vi "VFH-comp-libreVNAR140.vi"() -> ()   [LabVIEW 2020, in "VFH-VNA_File_Handler.lvlib"]
uses:
  VFH-VNA_File_Handler.lvlib
panel:
  out "Waveform Graph":dbl[][](graph)
  out "Raw 2":T1(graph)
  in  "r140":path=path "C:/projects/UNI/VNA/MiniVNA/20240625-162312-Vann/Vann.txt"
  out "Raw":T1(graph)
  in  "Libre":path=path "C:/projects/UNI/VNA/MiniVNA/20240625-162312-Vann/Vann.txt"
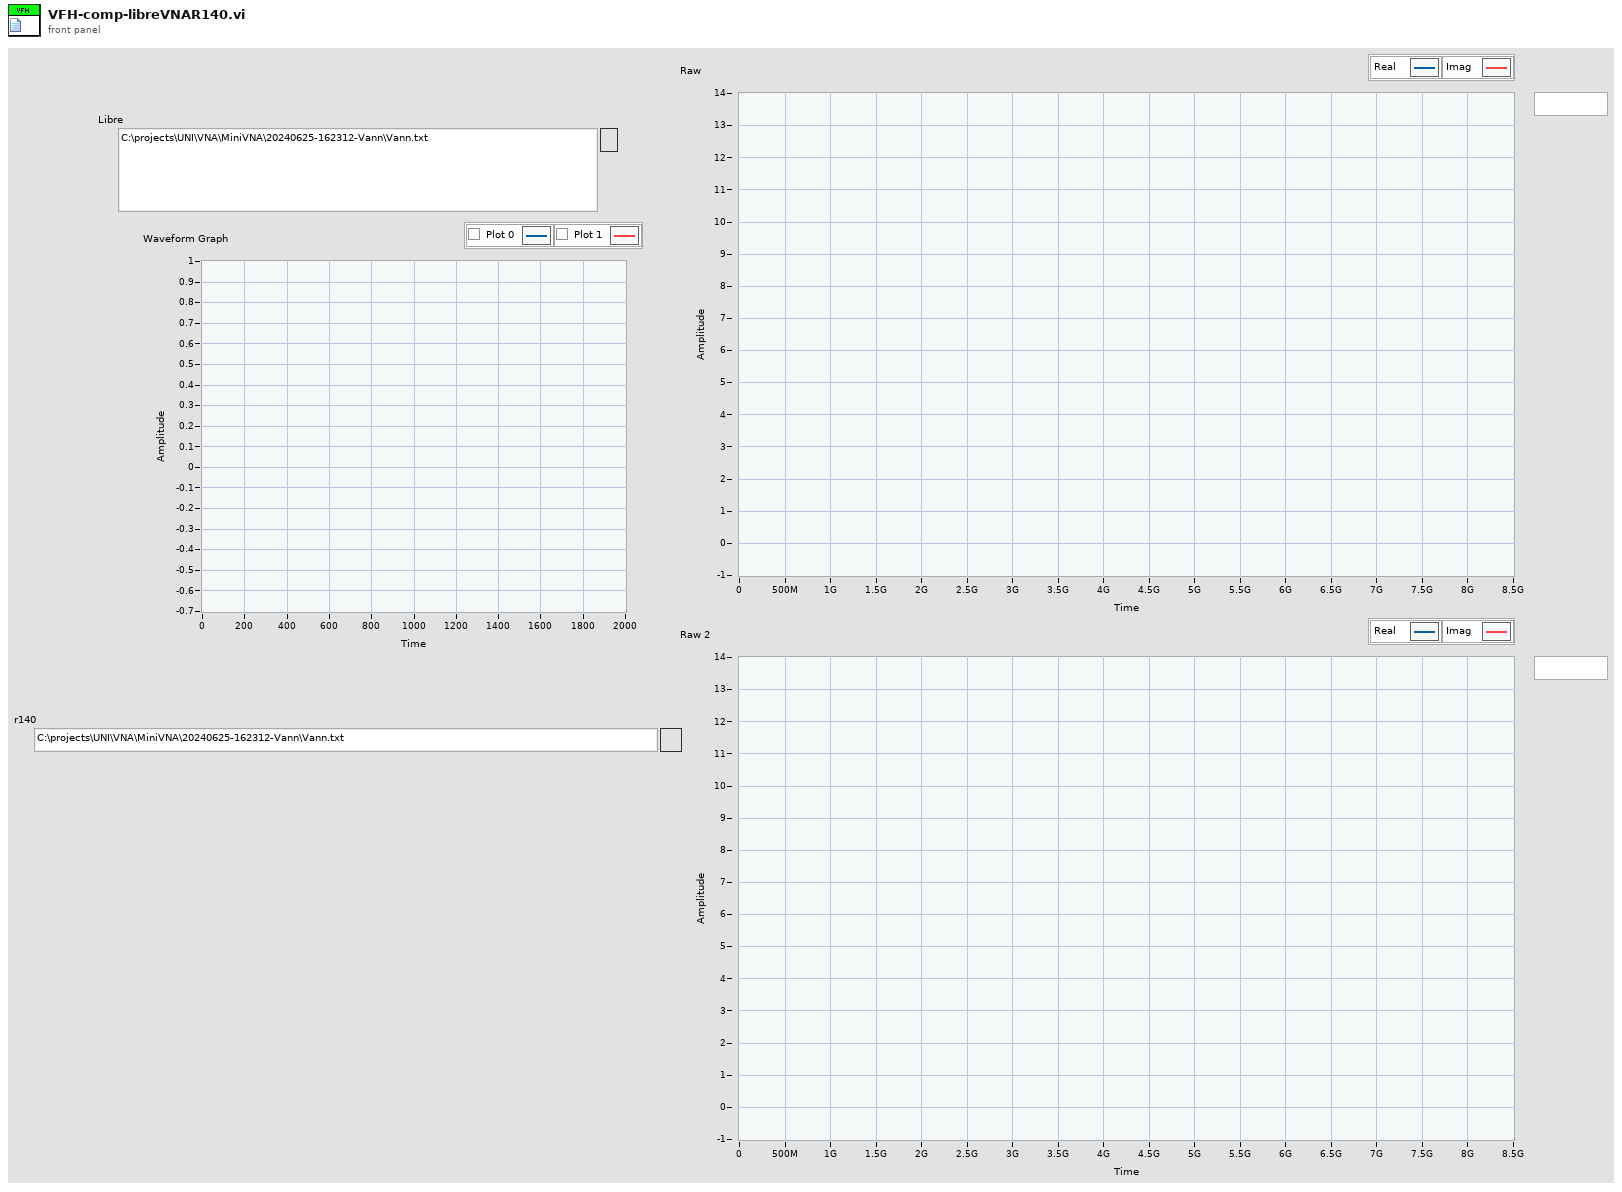
[diagram p1: front panel]
types:
  T1 = cluster{"Frequency":dbl[], "Reflection R":dbl[]}[]
  T2 = typedef "VFH-VNA_File_Handler.lvlib/VFH-file_cluster-R140.ctl" = cluster{"Frequency":dbl[], "Permativity'":dbl[], "Permativity''":dbl[], "Q [S/m]":dbl[], "Tan":dbl[], "Reflection R":dbl[], "Reflection I":dbl[]}
  T3 = typedef "VFH-VNA_File_Handler.lvlib/VFH-file_cluster-NanoVNA.ctl" = cluster{"Frequency":dbl[], "S11_Real":dbl[], "S11_Imag":dbl[], "S21_Real":dbl[], "S21_Imag":dbl[], "S12_Real":dbl[], "S12_Imag":dbl[], "S22_Real":dbl[], "S22_Imag":dbl[]}
  T4 = cluster{"Frequency":dbl[], "Reflection I":dbl[]}[]
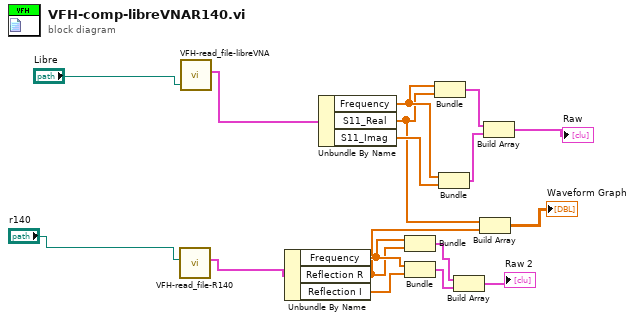
[diagram p0: block diagram]
diagram:
  n1 = call "VFH-read_file-R140.vi"("file path (dialog if empty)"="r140") -> ("output cluster"=w3:T2)  [unwired: 9 in, 1 out]
  n2 = call "VFH-read_file-libreVNA.vi"("file path (dialog if empty)"="Libre") -> ("output cluster"=w1:T3)  [unwired: 9 in, 1 out]
  n3 = Unbundle By Name(w3) -> ("Frequency"=w10:dbl[], "Reflection R"=w6:dbl[], "Reflection I"=w11:dbl[])
  n4 = Unbundle By Name(w1) -> ("Frequency"=w8:dbl[], "S11_Real"=w7:dbl[], "S11_Imag"=w17:dbl[])
  n5 = Bundle("Frequency"=w10, "Reflection R"=w6) -> (w9:cluster{"Frequency":dbl[], "Reflection R":dbl[]})  [unwired: 1 in]
  n6 = Bundle("Frequency"=w10, "Reflection I"=w11) -> (w12:cluster{"Frequency":dbl[], "Reflection I":dbl[]})  [unwired: 1 in]
  n7 = Bundle("Frequency"=w8, "S11_Real"=w7) -> (w16:cluster{"Frequency":dbl[], "S11_Real":dbl[]})  [unwired: 1 in]
  n8 = Bundle("Frequency"=w8, "S11_Imag"=w17) -> (w15:cluster{"Frequency":dbl[], "S11_Imag":dbl[]})  [unwired: 1 in]
  n9 = Build Array(w9, w12) -> (→"Raw 2":T4)
  n10 = Build Array(w7, w6) -> (→"Waveform Graph":dbl[][])
  n11 = Build Array(w16, w15) -> (→"Raw":cluster{"Frequency":dbl[], "S11_Imag":dbl[]}[])
